vi "Teleop.vi"(10 "Match Info":T5={"Autonomous Elapsed Seconds"=0.0, "TeleOp Elapsed Seconds"=0.0, "Disabled Elapsed Seconds"=0.0, "Visited Autonomous"=FALSE, "Visited TeleOp"=FALSE, "Visited Disabled"=FALSE, "Autonomous Settings"={"Autonomous Style"=enum."Independent", "VI Refnum"=refnum}}, 11 "Call Context":T6) -> ()   [LabVIEW 2017]
doc: "This VI is called for each TeleOp packet received from the DS where the robot is not disabled. It is often used to read from the joysticks and update I/O or to update setpoints for timed control loops. It should complete and return within 20 milliseconds or it may miss DS packets."
uses:
  <vilib>/Rock Robotics/WPI/DriverStation/WPI_DriverStationDerivedRobotMode.ctl
  <vilib>/Rock Robotics/WPI/DriverStation/WPI_DriverStationMatch Info.ctl
  <vilib>/Rock Robotics/WPI/ThirdParty/Sensors/navX/_TypeDefs/Flags/Z900_navX_Flags_OpStatusTypeDef.ctl
  <vilib>/Rock Robotics/WPI/ThirdParty/Sensors/navX/_TypeDefs/Flags/Z900_navX_Flags_CalibrationStatusTypeDef.ctl
  <vilib>/Rock Robotics/WPI/ThirdParty/Phoenix-LabVIEW/Motor Controller/Controls/CTRE_Phoenix_MotorControl_ControlMode.ctl
  <vilib>/Rock Robotics/WPI/Utilities/WPI_GetSetVariantRefNum.vi
  <vilib>/Rock Robotics/Network Tables/NT Write Boolean Array.vi
  <vilib>/Rock Robotics/Network Tables/NT Write Numeric Array.vi
  <vilib>/Rock Robotics/Network Tables/NT Read Boolean.vi
  <vilib>/Rock Robotics/Network Tables/NT Read Number.vi
panel:
  in  "Self Righting":bool
  out "lift":dbl
  in  "D Gain":dbl=0.0004 format="%#_13g"
  in  "P Gain":dbl=0.04 format="%#_13g"
  out "Status":T3 {"OP Status" items=["INITIALIZING", "SELFTEST_IN_PROGRESS", "ERROR", "IMU_AUTOCAL_IN_PROGRESS", "NORMAL"]; "Calibration Status" items=["IMU_CAL_STATE_MASK"=3, "IMU_CAL_STATE_INPROGRESS"=0, "IMU_CAL_STATE_ACCUMULATE"=1, "IMU_CAL_STATE_COMPLETE"=2]}
  out "YRPHfH":T4
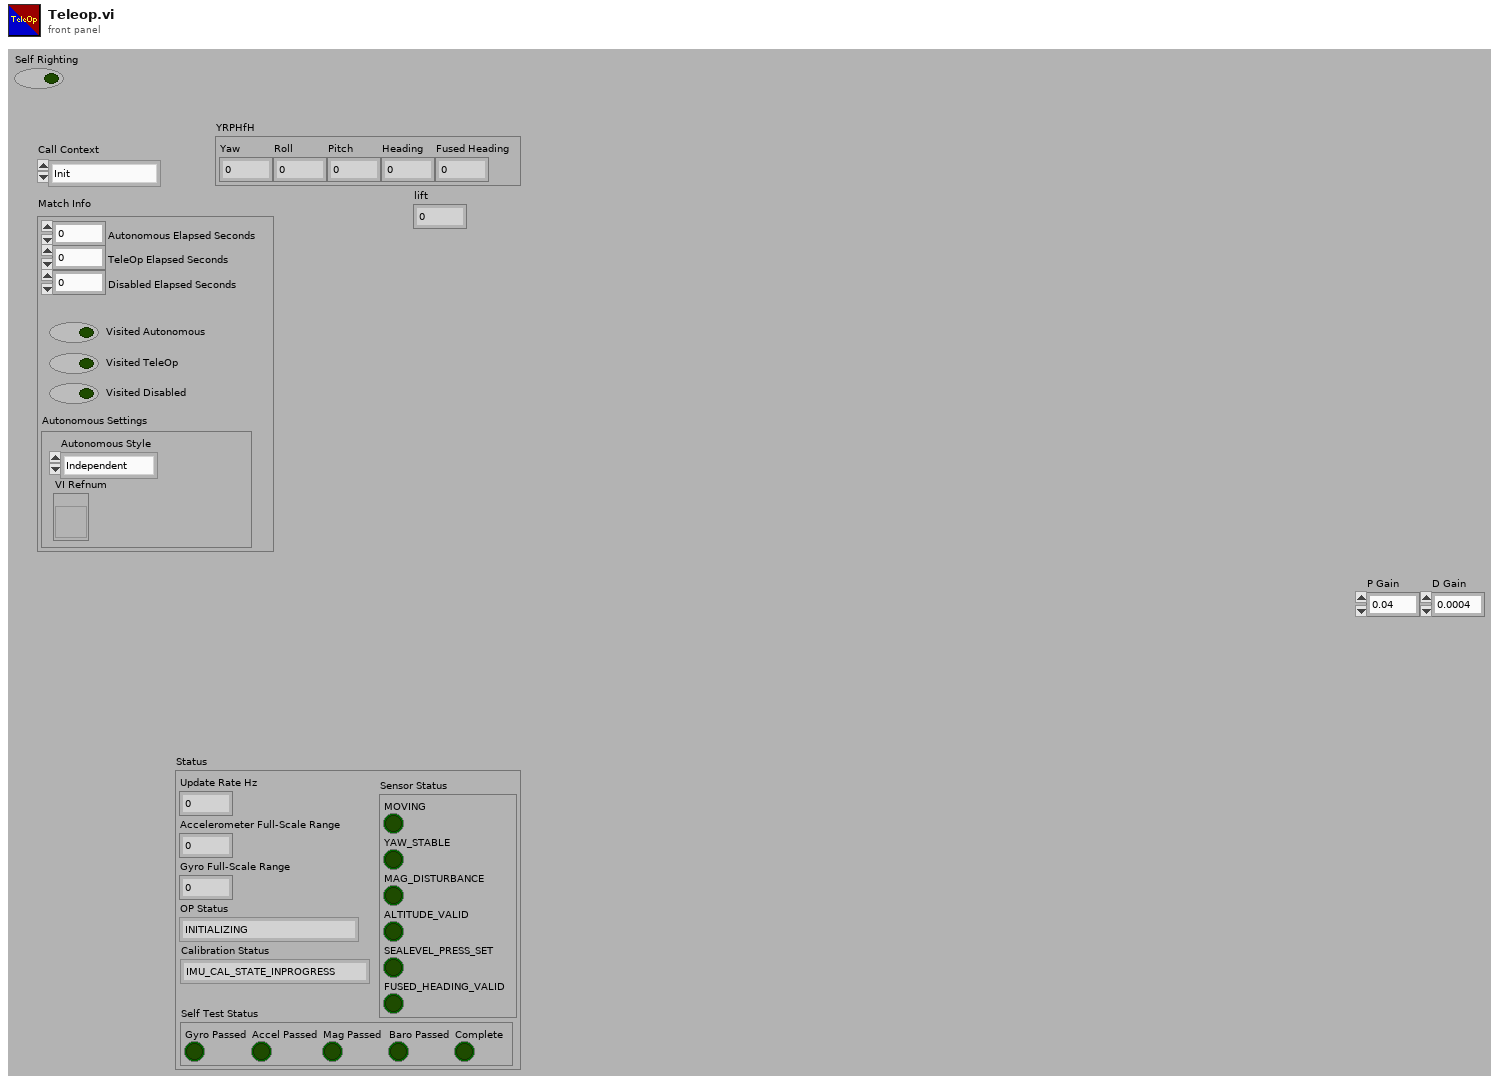
[diagram p1: front panel]
types:
  T1 = typedef "Z900_navX_Flags_OpStatusTypeDef.ctl" = u8
  T2 = typedef "Z900_navX_Flags_CalibrationStatusTypeDef.ctl" = u8
  T3 = cluster{"Update Rate Hz":u8, "Accelerometer Full-Scale Range":u8, "Gyro Full-Scale Range":u16, "OP Status":T1, "Calibration Status":T2, "Sensor Status":cluster{"MOVING":bool, "YAW_STABLE":bool, "MAG_DISTURBANCE":bool, "ALTITUDE_VALID":bool, "SEALEVEL_PRESS_SET":bool, "FUSED_HEADING_VALID":bool}, "Self Test Status":cluster{"Gyro Passed":bool, "Accel Passed":bool, "Mag Passed":bool, "Baro Passed":bool, "Complete":bool}}
  T4 = cluster{"Yaw":dbl, "Roll":dbl, "Pitch":dbl, "Heading":dbl, "Fused Heading":dbl}
  T5 = typedef "WPI_DriverStationMatch Info.ctl" = cluster{"Autonomous Elapsed Seconds":dbl, "TeleOp Elapsed Seconds":dbl, "Disabled Elapsed Seconds":dbl, "Visited Autonomous":bool, "Visited TeleOp":bool, "Visited Disabled":bool, "Autonomous Settings":cluster{"Autonomous Style":enum16{"Iterative", "Independent"}, "VI Refnum":refnum<vi>}}
  T6 = typedef "WPI_DriverStationDerivedRobotMode.ctl" = enum16{"Init", "Execute", "Stop"}
  T7 = typedef "CTRE_Phoenix_MotorControl_ControlMode.ctl" = u16
  T8 = typedef "WPI_JoystickDevRef.ctl" = cluster{"Device":T9}
  T9 = typedef "WPI_JoystickDeviceEnum.ctl" = enum16{"USB 0", "USB 1", "USB 2", "USB 3", "USB 4", "USB 5"}
  T10 = typedef "WPI_MotorControlDeviceRef.ctl" = cluster{"DeviceStatus":errorcluster, "Type":T11, "PWM":cluster{"PWM Channel":T12, "DeadBand":T13}, "CAN":cluster{"Device Number":u8, "SetOutput VI Ref":variant, "GetOutput VI Ref":variant, "Enable VI Ref":variant, "Disable VI Ref":variant, "Data":variant}, "Invert":bool, "DIO PWM":cluster{"PWM \"Enable\" Channel":T12, "DIOChannel":T14, "PWM Rate":dbl}}
  T11 = typedef "WPI_MotorControlType.ctl" = enum16{"PWM", "CAN", "DIO PWM"}
  T12 = typedef "FPGA_DIOPWMChannel.ctl" = enum8{"PWM 0", "PWM 1", "PWM 2", "PWM 3", "PWM 4", "PWM 5", "PWM 6", "PWM 7", "PWM 8", "PWM 9", "PWM MXP 0", "PWM MXP 1", "PWM MXP 2", "PWM MXP 3", "PWM MXP 4", "PWM MXP 5", "PWM MXP 6", "PWM MXP 7", "PWM MXP 8", "PWM MXP 9", "Invalid"}
  T13 = typedef "WPI_PWMDeadband.ctl" = cluster{"Name":string, "maxPositivePwm":i32, "minPositivePwm":i32, "centerPwm":i32, "maxNegativePwm":i32, "minNegativePwm":i32, "angularRange":u16}
  T14 = typedef "FPGA_DIOChannel.ctl" = enum8{"DIO 0", "DIO 1", "DIO 2", "DIO 3", "DIO 4", "DIO 5", "DIO 6", "DIO 7", "DIO 8", "DIO 9", "DIO MXP 0", "DIO MXP 1", "DIO MXP 2", "DIO MXP 3", "DIO MXP 4", "DIO MXP 5", "DIO MXP 6", "DIO MXP 7", "DIO MXP 8", "DIO MXP 9", "DIO MXP 10", "DIO MXP 11", "DIO MXP 12", "DIO MXP 13", "DIO MXP 14", "DIO MXP 15", "SPI Port CS1", "SPI Port CS2", "SPI Port CS3", "SPI Port MISO", "SPI Port MOSI", "Invalid"}
  T15 = typedef "WPI_RobotDriveDevRef.ctl" = cluster{"DevStatus":errorcluster, "Motors[]":T10[], "Square Inputs":bool, "Max Output":dbl}
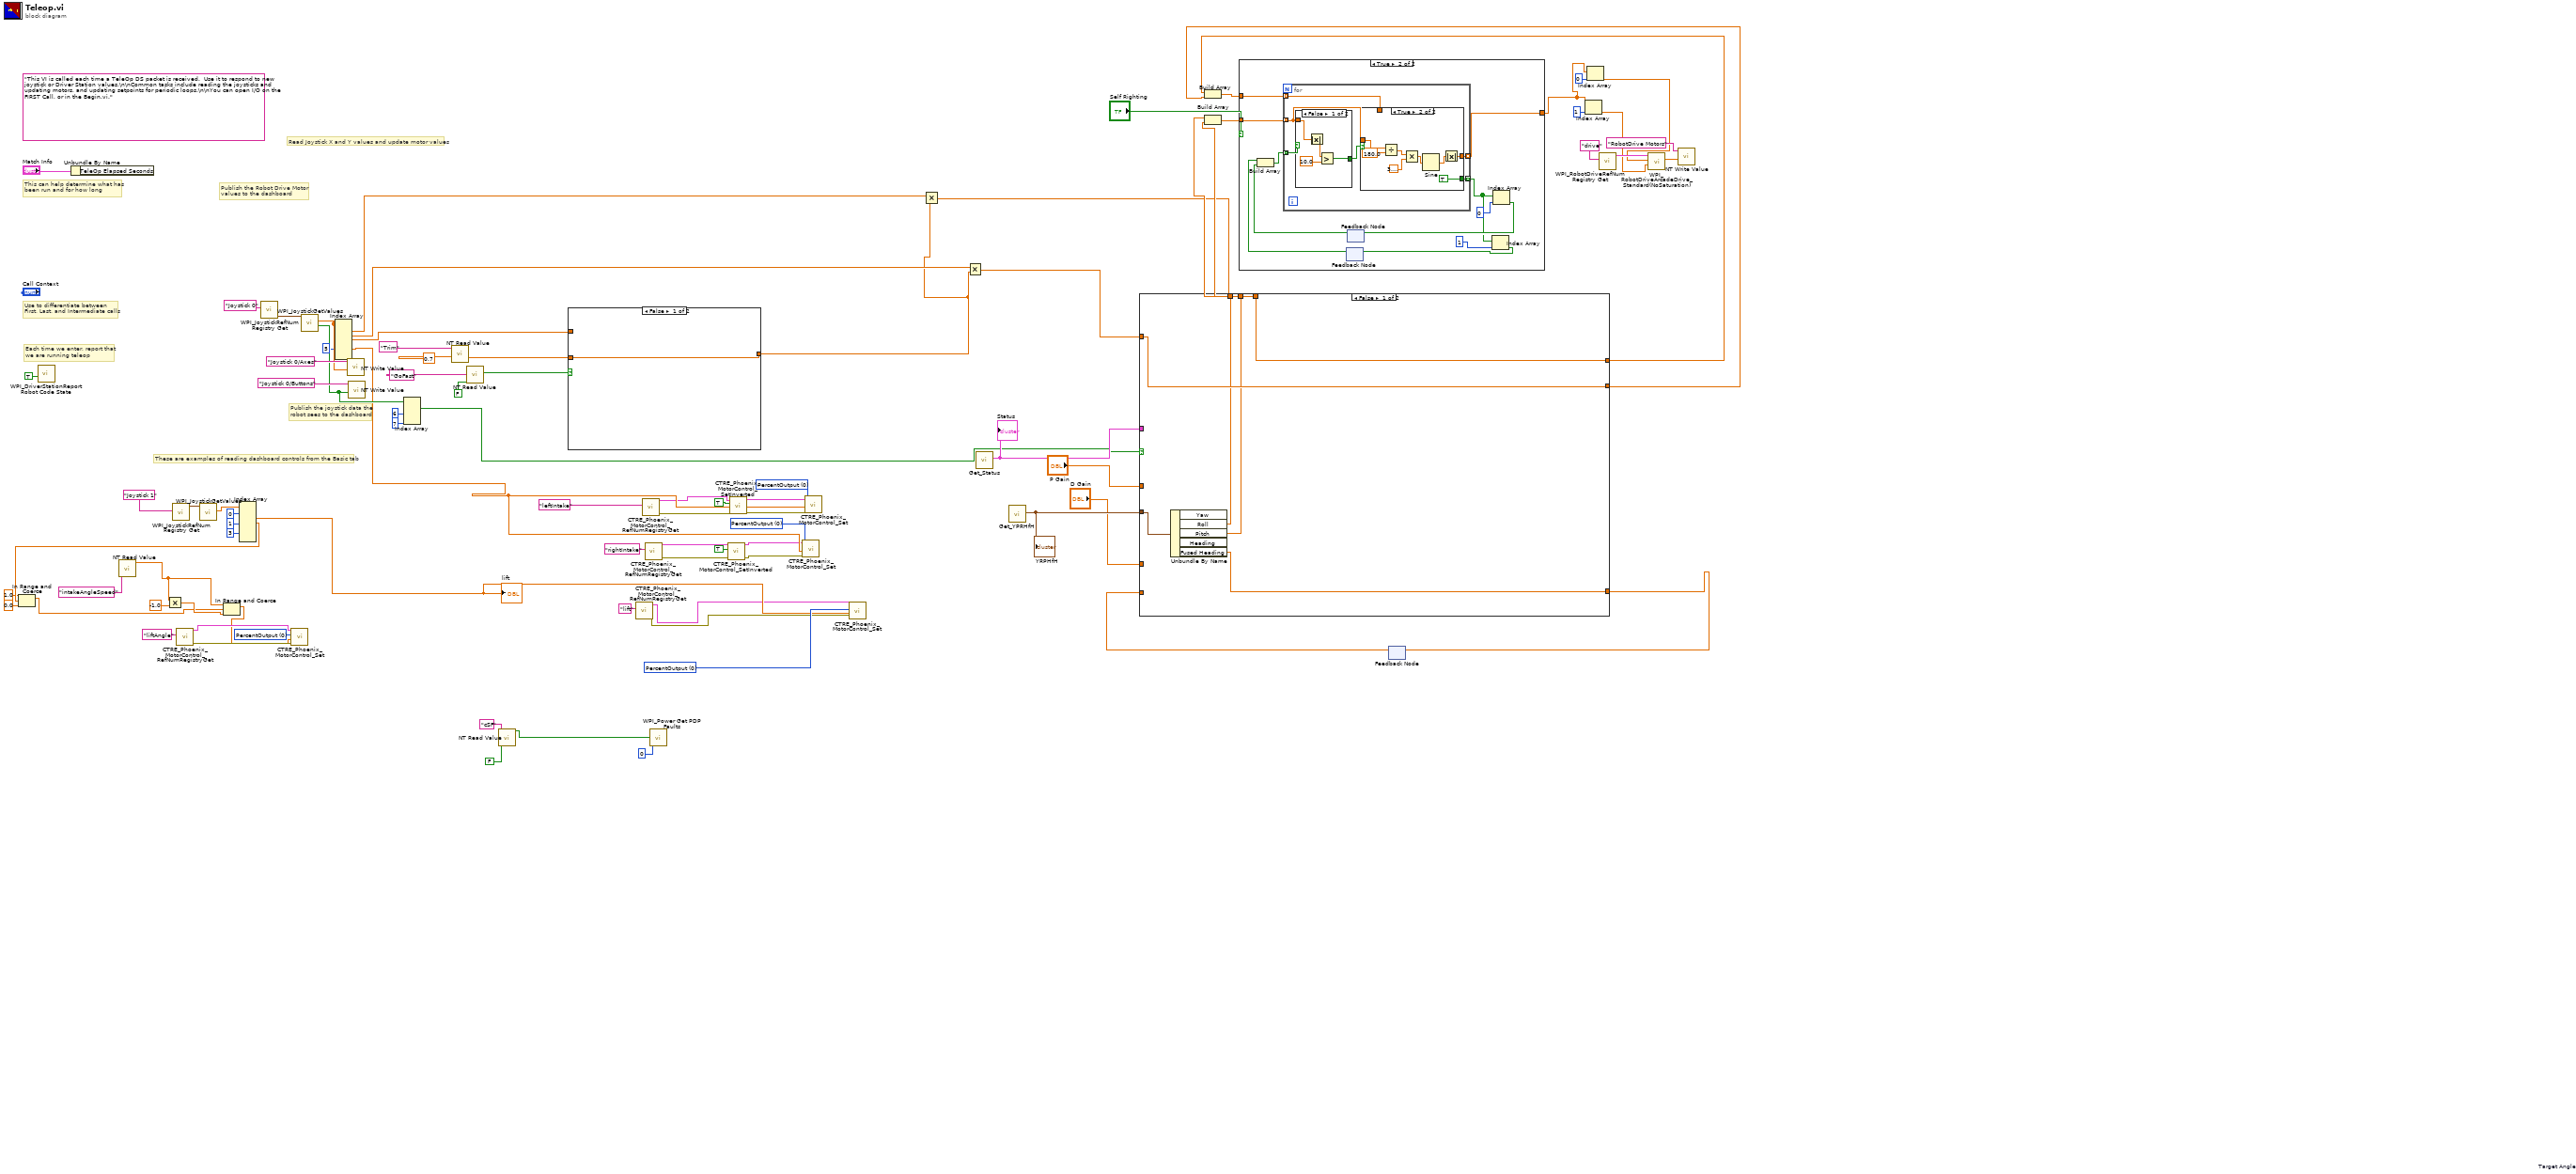
[diagram p0: block diagram]
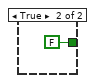
[diagram p4: hidden frame]
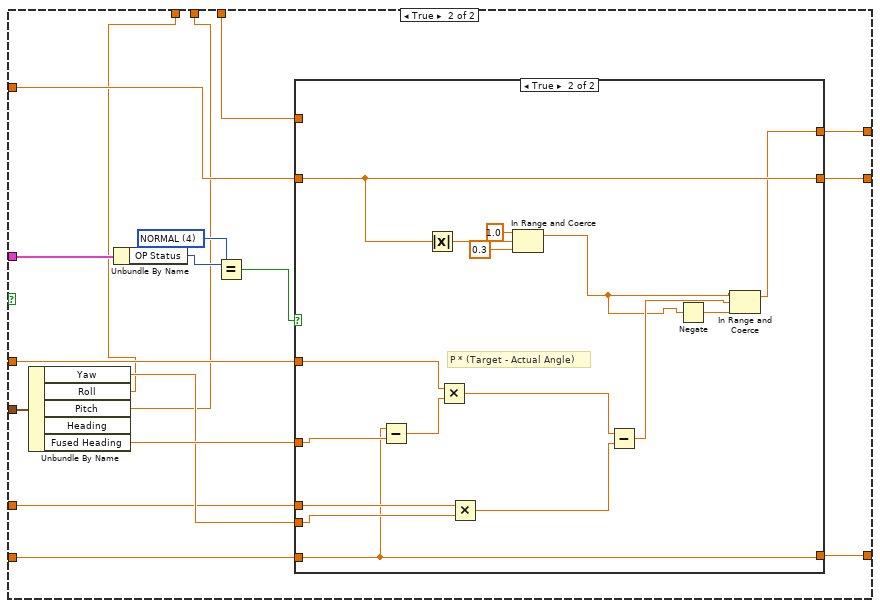
[diagram p5: hidden frame]
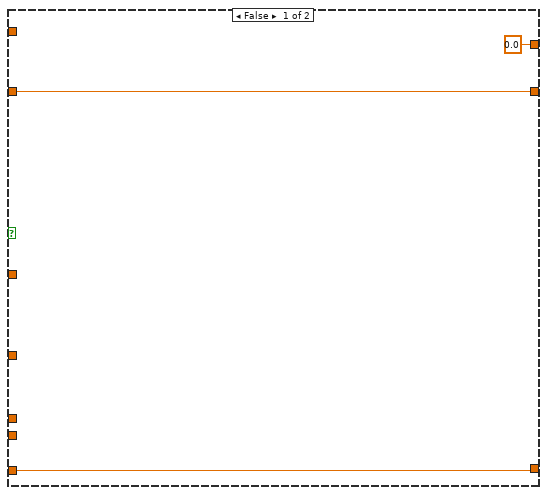
[diagram p6: hidden frame]
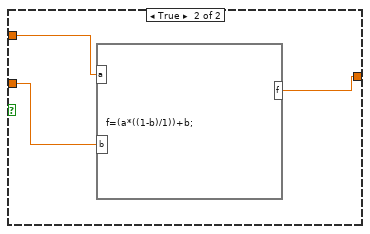
[diagram p7: hidden frame]
diagram:
  w30 = T7 0 items=["PercentOutput"=0, "Position"=1, "Velocity"=2, "Current"=3, "Follower"=5, "MotionProfile"=6, "MotionMagic"=7, "MotionMagicArc"=8, "MotionProfileArc"=10, "Disabled"=15] ("Control Mode")
  w32 = T7 0 items=["PercentOutput"=0, "Position"=1, "Velocity"=2, "Current"=3, "Follower"=5, "MotionProfile"=6, "MotionMagic"=7, "MotionMagicArc"=8, "MotionProfileArc"=10, "Disabled"=15] ("Control Mode")
  w33 = T7 0 items=["PercentOutput"=0, "Position"=1, "Velocity"=2, "Current"=3, "Follower"=5, "MotionProfile"=6, "MotionMagic"=7, "MotionMagicArc"=8, "MotionProfileArc"=10, "Disabled"=15] ("Control Mode")
  w43 = T7 0 items=["PercentOutput"=0, "Position"=1, "Velocity"=2, "Current"=3, "Follower"=5, "MotionProfile"=6, "MotionMagic"=7, "MotionMagicArc"=8, "MotionProfileArc"=10, "Disabled"=15] ("Control Mode")
  (unwired) "This VI is called each time a TeleOp DS packet is received.  Use it to respond to new joystick or Driver Station values.\n\nCommon tasks include reading the joysticks and updating motors, and updating setpoints for periodic loops.\n\nYou can open I/O on the FIRST Call, or in the Begin.vi."
  # "These are examples of reading dashboard controls from the Basic tab"
  # "Publish the Robot Drive Motor\nvalues to the dashboard"
  # "Publish the joystick data the\nrobot sees to the dashboard"
  # "Each time we enter, report that\nwe are running teleop"
  # "Use to differentiate between\nFirst, Last, and Intermediate calls"
  # "This can help determine what has\nbeen run and for how long"
  # "Read Joystick X and Y values and update motor values"
  n1 = call <vilib>:"WPI_DriverStationReport Robot Code State.vi"("TeleOp"=TRUE ("Autonomous")) -> ()  [unwired: 10 in, 1 out]
  n2 = Unbundle By Name("Match Info") -> ()  [unwired: 1 out]
  n3 = call-poly <vilib>:"NT Read Value.vi"("Name"="intakeAngleSpeed") -> ("Numeric"=w22:dbl)  [unwired: 9 in, 1 out]
  n4 = Multiply(x=w22, y=-1.0) -> (x*y=w20:dbl)
  n5 = call <vilib>:"WPI_JoystickRefNum Registry Get.vi"("refnum name"="Joystick 1") -> ("JoystickDevRef"=w39:T8)  [unwired: 1 in, 9 out]
  n6 = call <vilib>:"CTRE_Phoenix_MotorControl_RefNumRegistryGet.vi"("refnum name"="liftAngle") -> ("error out"=w25:errorcluster, "PhoenixMotorControlDevRef"=w26:T10)  [unwired: 9 in]
  n7 = call <vilib>:"WPI_JoystickGetValues.vi"("JoystickDevRef"=w39) -> ("Axes"=w38:dbl[])  [unwired: 6 in, 4 out]
  n8 = Index Array(array=w38, index #1=0 ("index"), index #2=1 ("index"), index #3=3 ("index")) -> (element #2=w28:dbl, element #3=w3:dbl)  [unwired: 4 in, 5 out]
  "lift" <- w28
  n9 = In Range and Coerce(upper limit=1.0, x=w3, lower limit=0.0) -> (coerced(x)=w4:dbl)  [unwired: 1 out]
  n10 = In Range and Coerce(upper limit=w22, x=w4, lower limit=w20) -> (coerced(x)=w24:dbl)  [unwired: 1 out]
  n11 = call <vilib>:"WPI_JoystickRefNum Registry Get.vi"("refnum name"="Joystick 0") -> ("JoystickDevRef"=w85:T8)  [unwired: 1 in, 9 out]
  n12 = call <vilib>:"CTRE_Phoenix_MotorControl_Set.vi"("error in (no error)"=w25, "Output"=w24, "Control Mode"=w30, "PhoenixMotorControlDevRef"=w26) -> ()  [unwired: 6 in, 2 out]
  n13 = call <vilib>:"WPI_JoystickGetValues.vi"("JoystickDevRef"=w85) -> ("Buttons"=w63:bool[], "Axes"=w81:dbl[])  [unwired: 6 in, 3 out]
  n14 = Index Array(array=w81, index #5=5 ("index")) -> (element #1=w70:dbl, element #2=w72:dbl, element #3=w59:dbl, element #5=w58:dbl)  [unwired: 6 in, 3 out]
  n15 = call-poly <vilib>:"NT Write Value.vi"("Numeric Array"=w81, "Name"="Joystick 0/Axes") -> ()  [unwired: 9 in, 1 out]
  n16 = call-poly <vilib>:"NT Write Value.vi"("Boolean Array"=w63, "Name"="Joystick 0/Buttons") -> ()  [unwired: 9 in, 1 out]
  n17 = Index Array(array=w63, index #2=6 ("index"), index #3=7 ("index")) -> (element #1=w62:bool)  [unwired: 2 in, 3 out]
  n18 = call-poly <vilib>:"NT Read Value.vi"("Default Value"=0.7, "Name"="Trim" ("refnum name")) -> ("Numeric"=w73:dbl)  [unwired: 8 in, 1 out]
  n19 = call-poly <vilib>:"NT Read Value.vi"("Default Value"=FALSE, "Name"="GoFast" ("refnum name")) -> ("Boolean"=w74:bool)  [unwired: 8 in, 1 out]
  n20 = call-poly <vilib>:"NT Read Value.vi"("Default Value"=FALSE, "Name"="cSF") -> ("Boolean"=w17:bool)  [unwired: 8 in, 1 out]
  n21 = case shown="False" w74 {
    tunnel: [w90 w93] -> w71
    tunnel: w73 -> [w90 w92]
    tunnel: w59 -> [_ w91]
    frame False {
    }
    frame True {
      n22 = formula code="f=(a*((1-b)/1))+b;"("a"=w91, "b"=w92) -> ("f"=w93:dbl)
    }
  }
  n23 = call <vilib>:"CTRE_Phoenix_MotorControl_RefNumRegistryGet.vi"("refnum name"="lift") -> ("error out"=w19:errorcluster, "PhoenixMotorControlDevRef"=w18:T10)  [unwired: 9 in]
  n24 = call <vilib>:"CTRE_Phoenix_MotorControl_RefNumRegistryGet.vi"("refnum name"="leftIntake") -> ("error out"=w12:errorcluster, "PhoenixMotorControlDevRef"=w13:T10)  [unwired: 9 in]
  n25 = call <vilib>:"CTRE_Phoenix_MotorControl_RefNumRegistryGet.vi"("refnum name"="rightIntake") -> ("error out"=w8:errorcluster, "PhoenixMotorControlDevRef"=w9:T10)  [unwired: 9 in]
  n26 = call <vilib>:"WPI_Power Get PDP Faults.vi"("Power Distribution Panel (0)"=u8 0, "Clear Sticky Faults"=w17) -> ()  [unwired: 9 in, 5 out]
  n27 = call <vilib>:"CTRE_Phoenix_MotorControl_SetInverted.vi"("error in (no error)"=w8, "Invert?"=TRUE, "PhoenixMotorControlDevRef"=w9) -> ("error out"=w6:errorcluster, "PhoenixMotorControlDevRef"=w7:T10)  [unwired: 7 in]
  n28 = call <vilib>:"CTRE_Phoenix_MotorControl_SetInverted.vi"("error in (no error)"=w12, "Invert?"=TRUE, "PhoenixMotorControlDevRef"=w13) -> ("error out"=w10:errorcluster, "PhoenixMotorControlDevRef"=w11:T10)  [unwired: 7 in]
  n29 = call <vilib>:"CTRE_Phoenix_MotorControl_Set.vi"("error in (no error)"=w6, "Output"=w58, "Control Mode"=w33, "PhoenixMotorControlDevRef"=w7) -> ()  [unwired: 6 in, 2 out]
  n30 = call <vilib>:"CTRE_Phoenix_MotorControl_Set.vi"("error in (no error)"=w10, "Output"=w58, "Control Mode"=w32, "PhoenixMotorControlDevRef"=w11) -> ()  [unwired: 6 in, 2 out]
  n31 = call <vilib>:"CTRE_Phoenix_MotorControl_Set.vi"("error in (no error)"=w19, "Output"=w28, "Control Mode"=w43, "PhoenixMotorControlDevRef"=w18) -> ()  [unwired: 6 in, 2 out]
  n32 = Multiply(x=w70, y=w71) -> (x*y=w48:dbl)
  n33 = Multiply(x=w72, y=w71) -> (x*y=w52:dbl)
  n34 = call <vilib>:"Get_Status.vi"() -> ("Status"=w68:T3)  [unwired: 11 in]
  "Status" <- w68
  n35 = call <vilib>:"Get_YPRHfH.vi"() -> ("YRPHfH"=w69:T4)  [unwired: 11 in]
  "YRPHfH" <- w69
  n36 = feedback #1 "Target Angle"() -> (w65:dbl)  [unwired: 1 in]
  n37 = case shown="False" w62 {
    tunnel: w69 -> [w97 w116]
    tunnel: w68 -> [_ w115]
    tunnel: "P Gain" -> [_ w109]
    tunnel: "D Gain" -> [_ w108]
    tunnel: w65 -> [_ w107]
    tunnel: w48 -> [w99 w106]
    tunnel: w52 -> [w98 w105]
    tunnel: [w98 w104] -> w46
    tunnel: [w99 w103] -> w47
    tunnel: [w96 w102] -> w64
    tunnel: [w95 w101] -> w51
    tunnel: [w94 w100] -> w50
    frame False {
      n38 = Unbundle By Name(w97) -> ("Roll"=w95:dbl, "Pitch"=w94:dbl, "Fused Heading"=w96:dbl)  [unwired: 2 out]
    }
    frame True {
      w113 = T1 4 items=["INITIALIZING", "SELFTEST_IN_PROGRESS", "ERROR", "IMU_AUTOCAL_IN_PROGRESS", "NORMAL"] ("y")
      n39 = Unbundle By Name(w116) -> ("Yaw"=w110:dbl, "Roll"=w101:dbl, "Pitch"=w100:dbl, "Fused Heading"=w111:dbl)  [unwired: 1 out]
      n40 = Unbundle By Name(w115) -> ("OP Status"=w114:T1)
      n41 = Equal?(x=w114, y=w113) -> (x = y?=w112:bool)
      n42 = case shown="True" w112 {
        tunnel: w111 -> [_ w135]
        tunnel: w110 -> [_ w132]
        tunnel: w109 -> [_ w133]
        tunnel: w108 -> [_ w131]
        tunnel: w107 -> [w119 w120]
        tunnel: w106 -> [_ _]
        tunnel: w105 -> [w118 w128]
        tunnel: [w118 w128] -> w104
        tunnel: [0.0 ("upper limit") w121] -> w103
        tunnel: [w119 w120] -> w102
        frame False {
        }
        frame True {
          # "P * (Target - Actual Angle)"
          n43 = Subtract(x=w120, y=w135) -> (x-y=w134:dbl)
          n44 = Absolute Value(x=w128) -> (abs(x)=w127:dbl)
          n45 = Multiply(x=w133, y=w134) -> (x*y=w130:dbl)
          n46 = Multiply(x=w131, y=w132) -> (x*y=w129:dbl)
          n47 = In Range and Coerce(upper limit=1.0, x=w127, lower limit=0.3) -> (coerced(x)=w122:dbl)  [unwired: 1 out]
          n48 = Subtract(x=w130, y=w129) -> (x-y=w124:dbl)
          n49 = Negate(x=w122) -> (-x=w123:dbl)
          n50 = In Range and Coerce(upper limit=w122, x=w124, lower limit=w123) -> (coerced(x)=w121:dbl)  [unwired: 1 out]
        }
      }
    }
  }
  n51 = Build Array(w47, w46) -> (w53:dbl[])
  n52 = Build Array(w51, w50) -> (w49:dbl[])
  n53 = case shown="True" "Self Righting" {
    tunnel: [w136 w147] -> w54
    tunnel: w53 -> [w136 w146]
    tunnel: w49 -> [_ w145]
    frame False {
    }
    frame True {
      n54 = feedback #2() -> (w140:bool)  [unwired: 1 in]
      n55 = feedback #3() -> (w141:bool)  [unwired: 1 in]
      n56 = Build Array(w140, w141) -> (w142:bool[])
      n57 = for {
        tunnel: [w153] -> w147 mode=indexing
        tunnel: w146 -> [w152] mode=indexing
        tunnel: w145 -> [w151] mode=indexing
        tunnel: [w150] -> w137 mode=indexing
        tunnel: w142 -> [w148] mode=indexing
        n58 = case shown="False" w148 {
          tunnel: w151 -> [w166 _]
          tunnel: [w164 FALSE] -> w149
          frame False {
            n59 = Absolute Value(x=w166) -> (abs(x)=w167:dbl)
            n60 = Greater?(x=w167, y=10.0) -> (0:w164:bool)
          }
          frame True {
          }
        }
        n61 = case shown="True" w149 {
          selector: w149 -> [w154 _]
          tunnel: [w155 w160] -> w153
          tunnel: w152 -> [w155 _]
          tunnel: w151 -> [_ w159]
          tunnel: [w154 TRUE] -> w150
          frame False {
          }
          frame True {
            n62 = Divide(x=w159, y=180.0) -> (x/y=w163:dbl)
            n63 = Multiply(x=w163, y=3.141592653589793) -> (x*y=w162:dbl)
            n64 = Sine(x=w162) -> (sin(x)=w161:dbl)
            n65 = Absolute Value(x=w161) -> (abs(x)=w160:dbl)
          }
        }
      }
      n66 = Index Array(array=w137, index=1) -> (element=w139:bool)
      n67 = feedback-in #2(w139) -> ()
      n68 = Index Array(array=w137, index=0) -> (element=w138:bool)
      n69 = feedback-in #3(w138) -> ()
    }
  }
  n70 = feedback-in #1(w64) -> ()
  n71 = Index Array(array=w54, index=1) -> (element=w45:dbl)
  n72 = Index Array(array=w54, index=0) -> (element=w44:dbl)
  n73 = call <vilib>:"WPI_RobotDriveRefNum Registry Get.vi"("refnum name"="drive") -> ("RobotDriveDevRef"=w87:T15)  [unwired: 1 in, 9 out]
  n74 = call <vilib>:"WPI_RobotDriveArcadeDrive_Standard(NoSaturation).vi"("Y axis value"=w45, "X axis value"=w44, "RobotDriveDevRef"=w87) -> ("Motor Values"=w80:dbl[])  [unwired: 1 in, 7 out]
  n75 = call-poly <vilib>:"NT Write Value.vi"("Numeric Array"=w80, "Name"="RobotDrive Motors") -> ()  [unwired: 9 in, 1 out]
